vi "getZkAndDofInGroups.vi"(8 "error in (no error)":errorcluster, 11 "ZTAAC in":refnum<class "ZTAAC.lvclass">) -> (0 "error out":errorcluster, 1 "DOF in Groups":T1, 2 "zn3Idx":bool[](array[boolean]), 3 "ZTAAC out":refnum<class "ZTAAC.lvclass">)   [LabVIEW 2016, in "OfcFunc.lvlib" / "ZTAAC.lvclass"]
doc: "Get the index array of Zk and DOF in groups (M2 hexapod, camera hexapod, M1M3 bending mode, M2 bending mode)."
uses:
  ZTAAC.lvclass
  ZTAAC.lvclass/ZTAAC.ctl
  OptStateEsti/OptStateEsti.lvclass
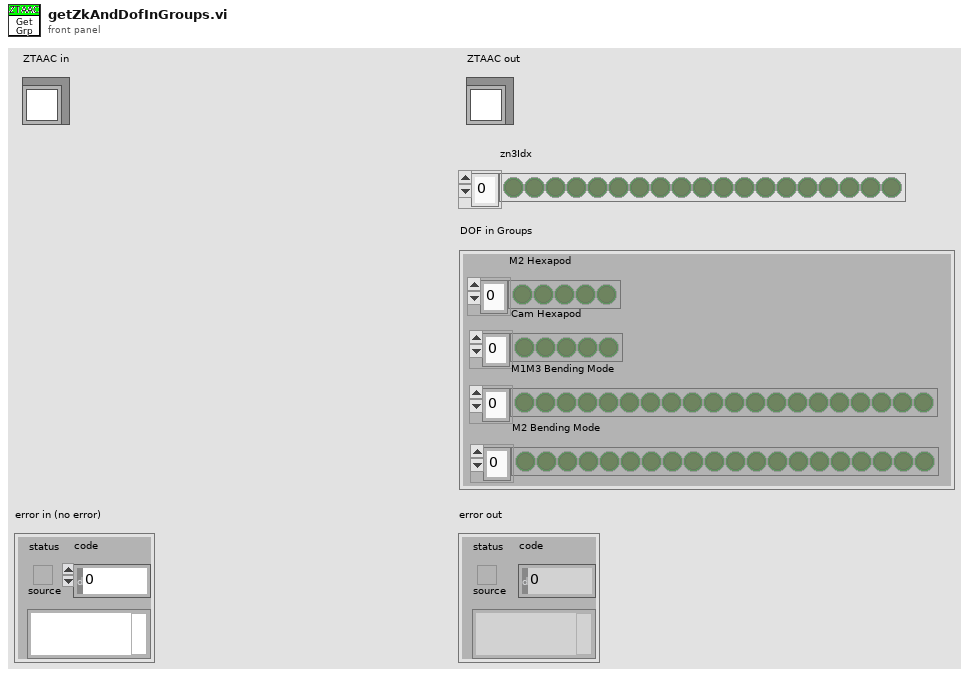
[diagram p1: front panel]
types:
  T1 = cluster{"M2 Hexapod":bool[], "Cam Hexapod ":bool[], "M1M3 Bending Mode":bool[], "M2 Bending Mode":bool[]}
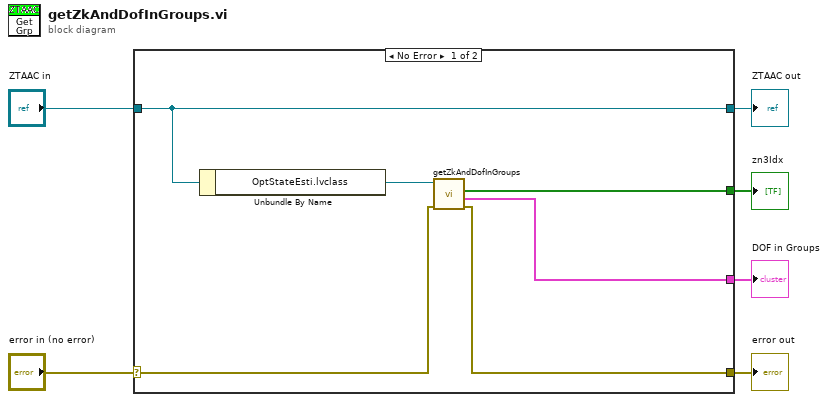
[diagram p0: block diagram]
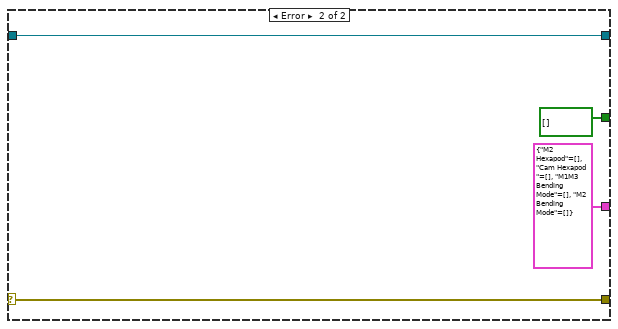
[diagram p2: hidden frame]
diagram:
  n1 = case shown="No Error" "error in (no error)" {
    selector: "error in (no error)" -> [w7 w16]
    tunnel: [w8 w16] -> w5
    tunnel: [w12 w15] -> w3
    tunnel: "ZTAAC in" -> [w12 w15]
    tunnel: [w10 bool[] [] ("zn3Idx")] -> w2
    tunnel: [w9 T1 {"M2 Hexapod"=[], "Cam Hexapod "=[], "M1M3 Bending Mode"=[], "M2 Bending Mode"=[]} ("DOF in Groups")] -> w1
    frame No Error {
      n2 = Unbundle By Name(w12) -> ("OptStateEsti.lvclass"=w11:refnum<class "OptStateEsti.lvclass">)
      n3 = call "getZkAndDofInGroups.vi"("error in (no error)"=w7, "OptStateEsti in"=w11) -> ("error out"=w8:errorcluster, "DOF in Groups"=w9:T1, "zn3Idx"=w10:bool[])  [unwired: 6 in, 1 out]
    }
    frame Error {
    }
  }
  "error out" <- w5
  "ZTAAC out" <- w3
  "zn3Idx" <- w2
  "DOF in Groups" <- w1
